vi "ReadParamBinFileFromControlProgram.vi"(0 "Array of Params (in format of control software parmas Typedef) in":T6[](array[typedef]) {"Instrument Calibr"."Psi" format="%#_2f"; "Manual Control"."Y peizo\n [nm]" scale=0.0..30000.0; "Manual Control"."AOM0 \nPower" scale=0.0..1.0; "Manual Control"."X piezo\n [nm]" scale=0.0..30000.0; "Manual Control"."Rotation Control"."freq difference [Hz]" step=0.5; "Manual Control"."Rotation Control"."mean freq  [MHz]\ndefault 39.99" min=0.0 step=0.01; "Manual Control"."Rotation Control"."B amp (0-120)" min=0.0 max=120.0 step=0.1; "Manual Control"."Rotation Control"."A amp (0-120)" min=0.0 max=120.0 step=0.1; "Manual Control"."Rotation Control"."Phase" scale=0.0..360.0; "Manual Control"."trap height\n [nm]" scale=1000.0..7500.0; "TaskIDs"."DAQ tasks"."Px taskID" format="%x"; "TaskIDs"."DAQ tasks"."Py taskID" format="%x"; "TaskIDs"."DAQ tasks"."Pz taskID" format="%x"; "TaskIDs"."DAQ tasks"."AOM taskID" format="%x"; "TaskIDs"."DAQ tasks"."Clock taskID" format="%x"; "TaskIDs"."DAQ tasks"."AI taskID" format="%x"}, 1 "file path in":path, 2 "Ignore HF and XYFTC calibration":bool, 3 "error in":errorcluster) -> (7 "Params out":T1={"Manual Control"={"Rotation Control"={"Phase"=0.0, "A amp (0-120)"=75.0, "B amp (0-120)"=53.3, "mean freq  [MHz]\ndefault 39.99"=40.0, "freq difference [Hz]"=2.0, "Enable A"=TRUE, "Enable B"=TRUE}, "X piezo\n [nm]"=0.0, "Y peizo\n [nm]"=0.0, "-Z piezo\n [nm]"=5.012658227848101, "AOM0 \nPower"=0.2}, "Piezo Calibr"={"Px2Vx(AO)"=nan, "Py2Vy(AO)"=nan, "Pz2Vz(AO)"=nan, "Min Px"=nan, "Min Py"=nan, "Min Pz"=nan, "Max Px"=nan, "Max Py"=nan, "Max Pz"=nan, "Vx0 (V)"=nan, "Vy0 (V)"=nan, "Vz0 (V)"=nan}, "Instrument Calibr"={"Angular compensation coeffs"=[], "TetherCenter"={"TrapX_AO 0 [nm]"=nan, "TrapY_AO 0 [nm]"=nan, "TrapZ_AO 0 [nm]"=nan}, "XYZsignal baseline"={"Xsignal0"=nan, "Ysignal0"=nan, "Zsignal0"=nan, "Zsig slope"=nan, "Z bead0"=nan}, "S and P to Vs0"={"Vs0/P"=1.0, "Vs0/S"=1.0}, "Psi"=0.0, "ePS:eRL drift correlation"={"Interc P"=nan, "Slope P"=nan, "Interc S"=nan, "Slope S"=nan}, "Current piezo volt AO"={"Vpx_AO [V]"=nan, "Vpy_AO [V]"=nan, "Vpz_AO [V]"=nan}}, "Cylinder Calibr"={"ZStiff"=nan, "Zsens"=nan, "AngStiff"=nan, "XStiff"=nan, "Xsens"=nan, "MaxEllip"=nan, "YStiff"=nan, "Ysens"=nan, "FocalShift"=nan, "Sfz"=nan, "1/Sz"=nan, "Stau"=nan, "Sfx"=nan, "1/Sx"=nan, "1/Sang"=nan, "Sfy"=nan, "1/Sy"=nan, "1/focal"=nan}, "DAQParams"={"Buffer size"=nan, "Scanning rate"=nan, "Average"=nan, "Sampling rate"=nan, "set dt"=nan}, "DAQ channel offsets"={"A0 [V]"=0.0, "D0 [V]"=0.0, "P0  [V]"=0.0, "S0 [V]"=0.0, "L0 [V]"=0.0, "R0 [V]"=0.0, "Vpx0 [V]"=0.0, "Vpy0 [V]"=0.0, "Vpz0 [V]"=0.0, "Vsum0 [V]"=0.0, "Vpx_AO0 [V]"=0.0, "Vpy_AO0 [V]"=0.0, "Vpz_AO0 [V]"=0.0}, "Z bead polynomial coeffs"=[nan, nan, nan, nan], "Skip button ref"=refnum, "z bead lookup table"={"z signal"=[], "z bead"=[]}, "SP->power Matrix"=[], "Ms2p"=[], "Mp2s"=[], "Polynomial coeff V_px,y,z 2 position (nm)"=[], "task in"=""} {"Instrument Calibr"."Psi" format="%#_2f"; "Manual Control"."Y peizo\n [nm]" scale=0.0..7000.0; "Manual Control"."AOM0 \nPower" scale=0.0..1.0; "Manual Control"."X piezo\n [nm]" scale=0.0..7000.0; "Manual Control"."Rotation Control"."freq difference [Hz]" step=0.5; "Manual Control"."Rotation Control"."mean freq  [MHz]\ndefault 39.99" min=0.0 step=0.01; "Manual Control"."Rotation Control"."B amp (0-120)" min=0.0 max=120.0 step=0.1; "Manual Control"."Rotation Control"."A amp (0-120)" min=0.0 max=120.0 step=0.1; "Manual Control"."Rotation Control"."Phase" scale=0.0..360.0; "Manual Control"."-Z piezo\n [nm]" scale=1000.0..7000.0}, 8 "file path out":path, 9 "Good?":bool, 10 "error out":errorcluster)   [LabVIEW 2017, in "Initialization.lvlib" / "FileManagement.lvlib"]
uses:
  FileManagement.lvlib
  Param_control program_170907.ctl
  <vilib>/Analysis/Matrix/Datatypes/RealMatrix.ctl
  New Param_170907.ctl
  ManualCtrl.ctl
  CylinderCalibrNew.ctl
  SignalConversion/DAQChannelOffsets.ctl
  <vilib>/Analysis/Matrix/NI_Matrix.lvlib
  Initialization.lvlib
  SignalConversion/SignalConverson.lvlib
panel:
  in  "Control software params as\nData type const":T6={"TaskIDs"={"DAQ tasks"={"Px taskID"=0, "Py taskID"=75, "Pz taskID"=53, "AOM taskID"=40, "Clock taskID"=2, "AI taskID"=0}, "DVEHandle"=refnum}, "Manual Control"={"Rotation Control"={"Phase"=0.0, "A amp (0-120)"=75.0, "B amp (0-120)"=53.3, "mean freq  [MHz]\ndefault 39.99"=40.0, "freq difference [Hz]"=2.0, "Enable A"=TRUE, "Enable B"=TRUE}, "X piezo\n [nm]"=nan, "Y peizo\n [nm]"=nan, "trap height\n [nm]"=nan, "AOM0 \nPower"=nan}, "Piezo Calibr"={"Px2Vx(AO)"=nan, "Py2Vy(AO)"=nan, "Pz2Vz(AO)"=nan, "Min Px"=nan, "Min Py"=0.0, "Min Pz"=nan, "Max Px"=nan, "Max Py"=nan, "Max Pz"=nan, "Vx0 (V)"=nan, "Vy0 (V)"=nan, "Vz0 (V)"=nan}, "Instrument Calibr"={"Angular compensation coeffs"=[], "TetherCenter"={"TrapX_AO 0 [nm]"=nan, "TrapY_AO 0 [nm]"=nan, "TrapZ_AO 0 [nm]"=nan}, "XYZsignal baseline"={"Xsignal0"=nan, "Ysignal0"=nan, "Zsignal0"=nan, "Zsig slope"=nan, "Z bead0"=nan}, "S and P to Vs0"={"Vs0/P"=1.0, "Vs0/S"=1.0}, "Psi"=nan, "ePS:eRL drift correlation"={"Interc P"=nan, "Slope P"=nan, "Interc S"=nan, "Slope S"=nan}, "Current piezo volt AO"={"Vpx_AO [V]"=nan, "Vpy_AO [V]"=nan, "Vpz_AO [V]"=nan}}, "Cylinder Calibr"={"ZStiff"=nan, "Zsens"=nan, "AngStiff"=nan, "XStiff"=nan, "Xsens"=nan, "MaxEllip"=nan, "YStiff"=nan, "Ysens"=nan, "FocalShift"=nan, "Sfz"=nan, "1/Sz"=nan, "Stau"=nan, "Sfx"=nan, "1/Sx"=nan, "1/Sang"=nan, "Sfy"=nan, "1/Sy"=nan, "1/focal"=nan}, "DAQParams"={"Buffer size"=0.0, "Scanning rate"=0.0, "Average"=0.0, "Sampling rate"=0.0, "set dt"=0.0}, "DAQ channel offsets"={"A0 [V]"=0.0, "D0 [V]"=0.0, "P0  [V]"=0.0, "S0 [V]"=0.0, "L0 [V]"=0.0, "R0 [V]"=0.0, "Vpx0 [V]"=0.0, "Vpy0 [V]"=0.0, "Vpz0 [V]"=0.0, "Vsum0 [V]"=0.0, "Vpx_AO0 [V]"=0.0, "Vpy_AO0 [V]"=0.0, "Vpz_AO0 [V]"=0.0}, "Z bead polynomial coeffs"=[nan, nan, nan, nan], "Skip button ref"=refnum, "z bead lookup table"={"z signal"=[], "z bead"=[]}, "SP->power Matrix"=[], "Ms2p"=[], "Mp2s"=[], "Polynomial coeff V_px,y,z 2 position (nm)"=[]} {"Instrument Calibr"."Psi" format="%#_2f"; "Manual Control"."Y peizo\n [nm]" scale=0.0..30000.0; "Manual Control"."AOM0 \nPower" scale=0.0..1.0; "Manual Control"."X piezo\n [nm]" scale=0.0..30000.0; "Manual Control"."Rotation Control"."freq difference [Hz]" step=0.5; "Manual Control"."Rotation Control"."mean freq  [MHz]\ndefault 39.99" min=0.0 step=0.01; "Manual Control"."Rotation Control"."B amp (0-120)" min=0.0 max=120.0 step=0.1; "Manual Control"."Rotation Control"."A amp (0-120)" min=0.0 max=120.0 step=0.1; "Manual Control"."Rotation Control"."Phase" scale=0.0..360.0; "Manual Control"."trap height\n [nm]" scale=1000.0..7500.0; "TaskIDs"."DAQ tasks"."Px taskID" format="%x"; "TaskIDs"."DAQ tasks"."Py taskID" format="%x"; "TaskIDs"."DAQ tasks"."Pz taskID" format="%x"; "TaskIDs"."DAQ tasks"."AOM taskID" format="%x"; "TaskIDs"."DAQ tasks"."Clock taskID" format="%x"; "TaskIDs"."DAQ tasks"."AI taskID" format="%x"}
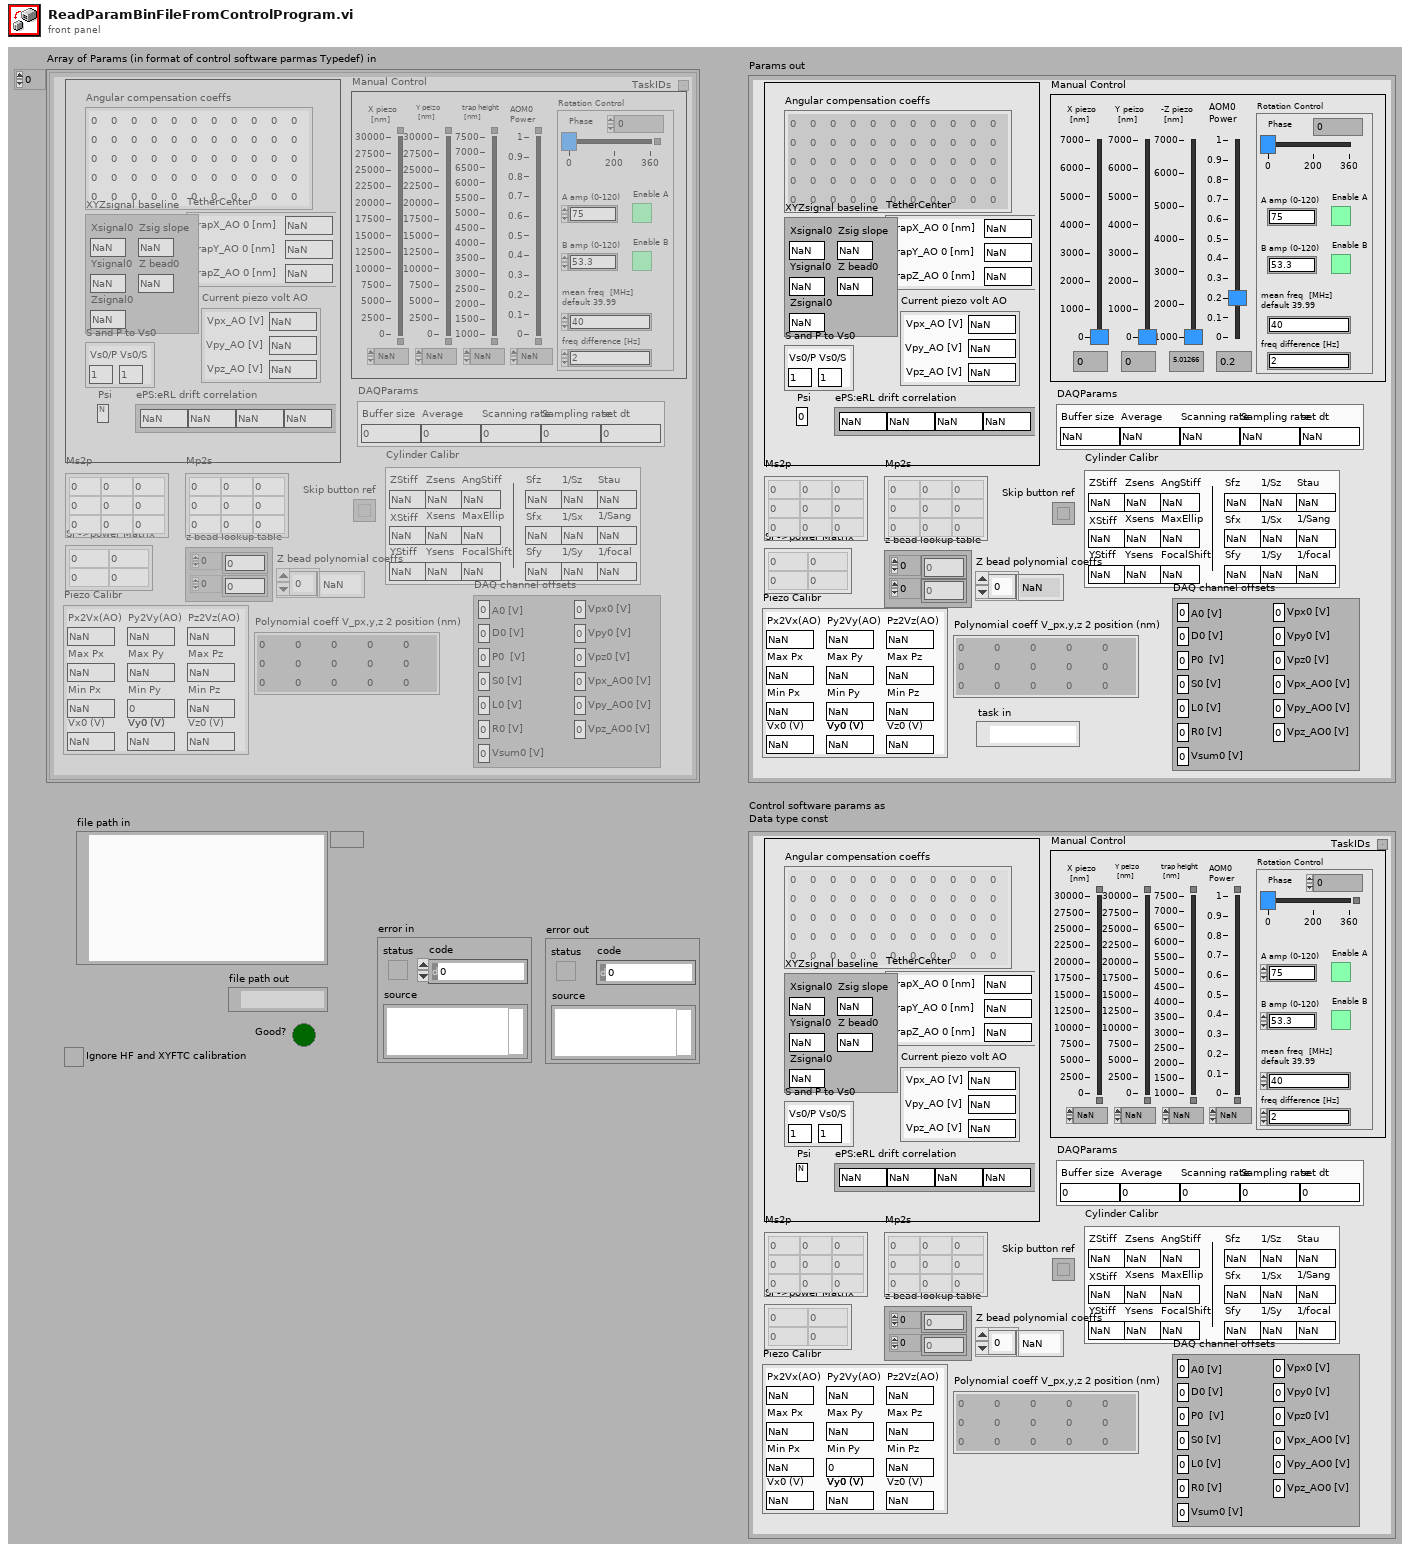
[diagram p1: front panel]
types:
  T1 = typedef "Initialization.lvlib/New Param_170907.ctl" = cluster{"Manual Control":T2, "Piezo Calibr":cluster{"Px2Vx(AO)":dbl, "Py2Vy(AO)":dbl, "Pz2Vz(AO)":dbl, "Min Px":dbl, "Min Py":dbl, "Min Pz":dbl, "Max Px":dbl, "Max Py":dbl, "Max Pz":dbl, "Vx0 (V)":dbl, "Vy0 (V)":dbl, "Vz0 (V)":dbl}, "Instrument Calibr":cluster{"Angular compensation coeffs":dbl[][], "TetherCenter":cluster{"TrapX_AO 0 [nm]":dbl, "TrapY_AO 0 [nm]":dbl, "TrapZ_AO 0 [nm]":dbl}, "XYZsignal baseline":cluster{"Xsignal0":dbl, "Ysignal0":dbl, "Zsignal0":dbl, "Zsig slope":dbl, "Z bead0":dbl}, "S and P to Vs0":cluster{"Vs0/P":dbl, "Vs0/S":dbl}, "Psi":dbl, "ePS:eRL drift correlation":cluster{"Interc P":dbl, "Slope P":dbl, "Interc S":dbl, "Slope S":dbl}, "Current piezo volt AO":cluster{"Vpx_AO [V]":dbl, "Vpy_AO [V]":dbl, "Vpz_AO [V]":dbl}}, "Cylinder Calibr":T3, "DAQParams":cluster{"Buffer size":dbl, "Scanning rate":dbl, "Average":dbl, "Sampling rate":dbl, "set dt":dbl}, "DAQ channel offsets":T4, "Z bead polynomial coeffs":dbl[], "Skip button ref":refnum<vi>, "z bead lookup table":cluster{"z signal":dbl[], "z bead":dbl[]}, "SP->power Matrix":T5, "Ms2p":T5, "Mp2s":T5, "Polynomial coeff V_px,y,z 2 position (nm)":dbl[][], "task in":refnum<k21>}
  T2 = typedef "Initialization.lvlib/ManualCtrl.ctl" = cluster{"Rotation Control":cluster{"Phase":dbl, "A amp (0-120)":dbl, "B amp (0-120)":dbl, "mean freq  [MHz]\ndefault 39.99":dbl, "freq difference [Hz]":dbl, "Enable A":bool, "Enable B":bool}, "X piezo\n [nm]":dbl, "Y peizo\n [nm]":dbl, "-Z piezo\n [nm]":dbl, "AOM0 \nPower":dbl}
  T3 = typedef "Initialization.lvlib/CylinderCalibrNew.ctl" = cluster{"ZStiff":dbl, "Zsens":dbl, "AngStiff":dbl, "XStiff":dbl, "Xsens":dbl, "MaxEllip":dbl, "YStiff":dbl, "Ysens":dbl, "FocalShift":dbl, "Sfz":dbl, "1/Sz":dbl, "Stau":dbl, "Sfx":dbl, "1/Sx":dbl, "1/Sang":dbl, "Sfy":dbl, "1/Sy":dbl, "1/focal":dbl}
  T4 = typedef "SignalConverson.lvlib/DAQChannelOffsets.ctl" = cluster{"A0 [V]":dbl, "D0 [V]":dbl, "P0  [V]":dbl, "S0 [V]":dbl, "L0 [V]":dbl, "R0 [V]":dbl, "Vpx0 [V]":dbl, "Vpy0 [V]":dbl, "Vpz0 [V]":dbl, "Vsum0 [V]":dbl, "Vpx_AO0 [V]":dbl, "Vpy_AO0 [V]":dbl, "Vpz_AO0 [V]":dbl}
  T5 = typedef "NI_Matrix.lvlib/RealMatrix.ctl" = dbl[][]
  T6 = typedef "Initialization.lvlib/Param_control program_170907.ctl" = cluster{"TaskIDs":cluster{"DAQ tasks":cluster{"Px taskID":u32, "Py taskID":u32, "Pz taskID":u32, "AOM taskID":u32, "Clock taskID":u32, "AI taskID":u32}, "DVEHandle":refnum<file>}, "Manual Control":cluster{"Rotation Control":cluster{"Phase":dbl, "A amp (0-120)":dbl, "B amp (0-120)":dbl, "mean freq  [MHz]\ndefault 39.99":dbl, "freq difference [Hz]":dbl, "Enable A":bool, "Enable B":bool}, "X piezo\n [nm]":dbl, "Y peizo\n [nm]":dbl, "trap height\n [nm]":dbl, "AOM0 \nPower":dbl}, "Piezo Calibr":cluster{"Px2Vx(AO)":dbl, "Py2Vy(AO)":dbl, "Pz2Vz(AO)":dbl, "Min Px":dbl, "Min Py":dbl, "Min Pz":dbl, "Max Px":dbl, "Max Py":dbl, "Max Pz":dbl, "Vx0 (V)":dbl, "Vy0 (V)":dbl, "Vz0 (V)":dbl}, "Instrument Calibr":cluster{"Angular compensation coeffs":dbl[][], "TetherCenter":cluster{"TrapX_AO 0 [nm]":dbl, "TrapY_AO 0 [nm]":dbl, "TrapZ_AO 0 [nm]":dbl}, "XYZsignal baseline":cluster{"Xsignal0":dbl, "Ysignal0":dbl, "Zsignal0":dbl, "Zsig slope":dbl, "Z bead0":dbl}, "S and P to Vs0":cluster{"Vs0/P":dbl, "Vs0/S":dbl}, "Psi":dbl, "ePS:eRL drift correlation":cluster{"Interc P":dbl, "Slope P":dbl, "Interc S":dbl, "Slope S":dbl}, "Current piezo volt AO":cluster{"Vpx_AO [V]":dbl, "Vpy_AO [V]":dbl, "Vpz_AO [V]":dbl}}, "Cylinder Calibr":cluster{"ZStiff":dbl, "Zsens":dbl, "AngStiff":dbl, "XStiff":dbl, "Xsens":dbl, "MaxEllip":dbl, "YStiff":dbl, "Ysens":dbl, "FocalShift":dbl, "Sfz":dbl, "1/Sz":dbl, "Stau":dbl, "Sfx":dbl, "1/Sx":dbl, "1/Sang":dbl, "Sfy":dbl, "1/Sy":dbl, "1/focal":dbl}, "DAQParams":cluster{"Buffer size":dbl, "Scanning rate":dbl, "Average":dbl, "Sampling rate":dbl, "set dt":dbl}, "DAQ channel offsets":cluster{"A0 [V]":dbl, "D0 [V]":dbl, "P0  [V]":dbl, "S0 [V]":dbl, "L0 [V]":dbl, "R0 [V]":dbl, "Vpx0 [V]":dbl, "Vpy0 [V]":dbl, "Vpz0 [V]":dbl, "Vsum0 [V]":dbl, "Vpx_AO0 [V]":dbl, "Vpy_AO0 [V]":dbl, "Vpz_AO0 [V]":dbl}, "Z bead polynomial coeffs":dbl[], "Skip button ref":refnum<vi>, "z bead lookup table":cluster{"z signal":dbl[], "z bead":dbl[]}, "SP->power Matrix":T5, "Ms2p":T5, "Mp2s":T5, "Polynomial coeff V_px,y,z 2 position (nm)":dbl[][]}
  T7 = enum16{"open", "replace", "create", "open or create", "replace or create", "replace or create with confirmation"}
  T8 = cluster{"Rotation Control":cluster{"Phase":dbl, "A amp (0-120)":dbl, "B amp (0-120)":dbl, "mean freq  [MHz]\ndefault 39.99":dbl, "freq difference [Hz]":dbl, "Enable A":bool, "Enable B":bool}, "X piezo\n [nm]":dbl, "Y peizo\n [nm]":dbl, "trap height\n [nm]":dbl, "AOM0 \nPower":dbl}
  T9 = cluster{"Px2Vx(AO)":dbl, "Py2Vy(AO)":dbl, "Pz2Vz(AO)":dbl, "Min Px":dbl, "Min Py":dbl, "Min Pz":dbl, "Max Px":dbl, "Max Py":dbl, "Max Pz":dbl, "Vx0 (V)":dbl, "Vy0 (V)":dbl, "Vz0 (V)":dbl}
  T10 = cluster{"Angular compensation coeffs":dbl[][], "TetherCenter":cluster{"TrapX_AO 0 [nm]":dbl, "TrapY_AO 0 [nm]":dbl, "TrapZ_AO 0 [nm]":dbl}, "XYZsignal baseline":cluster{"Xsignal0":dbl, "Ysignal0":dbl, "Zsignal0":dbl, "Zsig slope":dbl, "Z bead0":dbl}, "S and P to Vs0":cluster{"Vs0/P":dbl, "Vs0/S":dbl}, "Psi":dbl, "ePS:eRL drift correlation":cluster{"Interc P":dbl, "Slope P":dbl, "Interc S":dbl, "Slope S":dbl}, "Current piezo volt AO":cluster{"Vpx_AO [V]":dbl, "Vpy_AO [V]":dbl, "Vpz_AO [V]":dbl}}
  T11 = cluster{"ZStiff":dbl, "Zsens":dbl, "AngStiff":dbl, "XStiff":dbl, "Xsens":dbl, "MaxEllip":dbl, "YStiff":dbl, "Ysens":dbl, "FocalShift":dbl, "Sfz":dbl, "1/Sz":dbl, "Stau":dbl, "Sfx":dbl, "1/Sx":dbl, "1/Sang":dbl, "Sfy":dbl, "1/Sy":dbl, "1/focal":dbl}
  T12 = cluster{"Buffer size":dbl, "Scanning rate":dbl, "Average":dbl, "Sampling rate":dbl, "set dt":dbl}
  T13 = cluster{"A0 [V]":dbl, "D0 [V]":dbl, "P0  [V]":dbl, "S0 [V]":dbl, "L0 [V]":dbl, "R0 [V]":dbl, "Vpx0 [V]":dbl, "Vpy0 [V]":dbl, "Vpz0 [V]":dbl, "Vsum0 [V]":dbl, "Vpx_AO0 [V]":dbl, "Vpy_AO0 [V]":dbl, "Vpz_AO0 [V]":dbl}
  T14 = cluster{"TrapX_AO 0 [nm]":dbl, "TrapY_AO 0 [nm]":dbl, "TrapZ_AO 0 [nm]":dbl}
  T15 = cluster{"Xsignal0":dbl, "Ysignal0":dbl, "Zsignal0":dbl, "Zsig slope":dbl, "Z bead0":dbl}
  T16 = cluster{"Interc P":dbl, "Slope P":dbl, "Interc S":dbl, "Slope S":dbl}
  T17 = cluster{"Vpx_AO [V]":dbl, "Vpy_AO [V]":dbl, "Vpz_AO [V]":dbl}
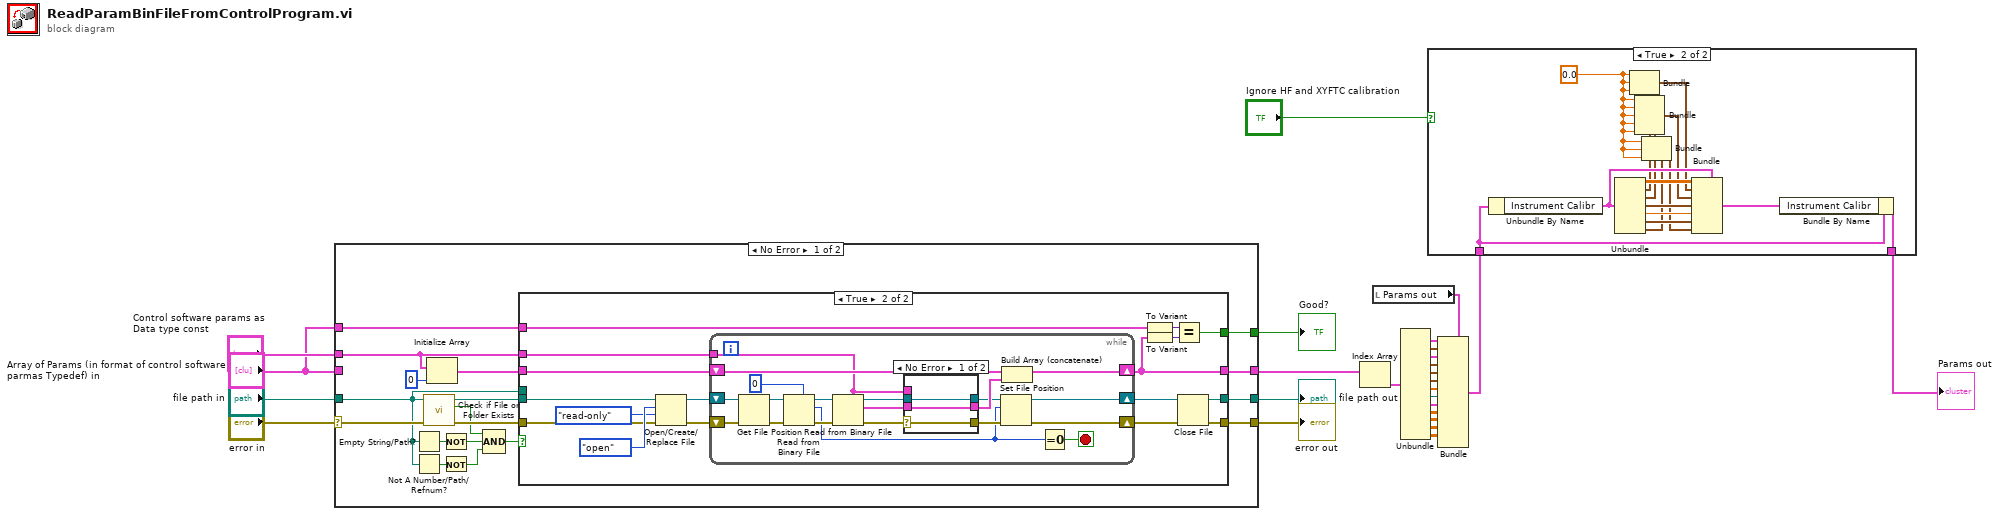
[diagram p0: block diagram]
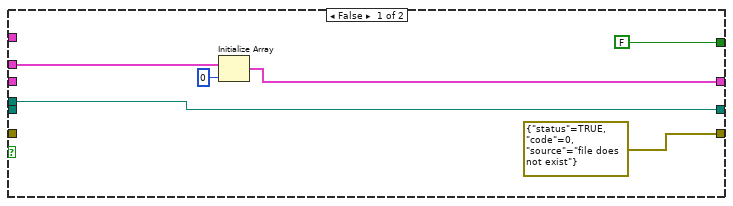
[diagram p3: hidden frame]
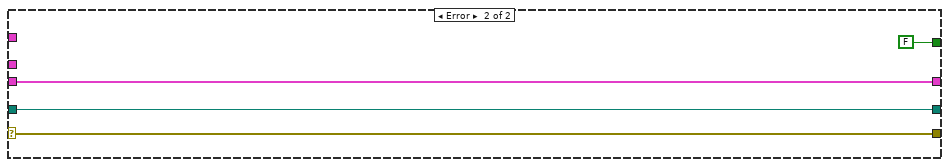
[diagram p5: hidden frame]
diagram:
  n1 = case shown="No Error" "error in" {
    selector: "error in" -> [w38 w96]
    tunnel: "file path in" -> [w31 w95]
    tunnel: "Array of Params (in format of control software parmas Typedef) in" -> [_ w94]
    tunnel: [w44 w96] -> w26
    tunnel: [w43 w95] -> w25
    tunnel: [w42 w94] -> w19
    tunnel: "Control software params as\nData type const" -> [w41 _]
    tunnel: "Array of Params (in format of control software parmas Typedef) in" -> [w40 _]
    tunnel: [w39 FALSE] -> w23
    frame No Error {
      n2 = Empty String/Path?(string/path=w31) -> (empty?=w33:bool)
      n3 = Not A Number/Path/Refnum?(number/path/refnum=w31) -> (NaN/Path/Refnum?=w32:bool)
      n4 = call <vilib>:"Check if File or Folder Exists.vi"("error in (no error)"=w38, "path"=w31) -> ("error out"=w34:errorcluster, "file or folder exists?"=w29:bool, "dup path"=w35:path)  [unwired: 7 in]
      n5 = Initialize Array(w41, 0 ("dimension size")) -> (w36:T6[])
      n6 = Not(x=w33) -> (.not. x?=w28:bool)
      n7 = Not(x=w32) -> (.not. x?=w27:bool)
      n8 = Compound Arithmetic op=AND(w29, w28, w27) -> (w30:bool)
      n9 = case shown="True" w30 {
        tunnel: [w48 w63] -> w42
        tunnel: w41 -> [w49 w67]
        tunnel: [w45 w58] -> w43
        tunnel: [errorcluster {"status"=TRUE, "code"=0, "source"="file does not exist"} ("error out") w59] -> w44
        tunnel: w36 -> [_ w66]
        tunnel: w40 -> [_ w62]
        tunnel: [FALSE w61] -> w39
        tunnel: w31 -> [w45 _]
        tunnel: w35 -> [_ w52]
        tunnel: w34 -> [_ w51]
        frame False {
          n10 = Initialize Array(w49, 0 ("dimension size")) -> (w48:T6[])
        }
        frame True {
          n11 = Open/Create/Replace File(file path (use dialog)=w52, error in=w51, operation (0:open)=T7."open", access (0:read/write)=enum16{"read/write", "read-only", "write-only"}."read-only") -> (refnum out=w53:refnum<file>, error out=w54:errorcluster)  [unwired: 2 in, 1 out]
          n12 = while {
            shift-right: [w86] -> w63
            shift-left: w66 -> [w84]
            tunnel: w67 -> [w69]
            shift-right: [w73] -> w57
            shift-left: w53 -> [w78]
            shift-right: [w72] -> w60
            shift-left: w54 -> [w81]
            stop <- w87 stop-if-true
            n13 = Get File Position(4:w81, 7:w78) -> (0:w80:errorcluster, 3:w79:refnum<file>)  [unwired: 1 out]
            n14 = Read from Binary File(5:i64 0, 8:w80, 11:w79) -> (0:w82:errorcluster, 2:w68:i64, 3:w83:refnum<file>)  [unwired: 3 in, 1 out]
            n15 = Read from Binary File(5:w69, 8:w82, 11:w83) -> (0:w76:errorcluster, 2:w75:T6, 3:w77:refnum<file>)  [unwired: 3 in, 1 out]
            n16 = case shown="No Error" w76 {
              selector: w76 -> [w89 _]
              tunnel: w77 -> [w88 w91]
              tunnel: w75 -> [w90 _]
              tunnel: [w90 w92] -> w74
              tunnel: [w89 _] -> w71
              tunnel: [w88 w91] -> w70
              tunnel: w69 -> [_ w92]
              frame No Error {
              }
              frame Error {
              }
            }
            n17 = Set File Position(offset (in bytes) (0)=w68, refnum=w70, error in=w71) -> (refnum out=w73:refnum<file>, error out=w72:errorcluster)  [unwired: 1 in]
            n18 = Build Array (concatenate)(w84, w74) -> (w86:T6[])
            n19 = Equal To 0?(x=w68) -> (x = 0?=w87:bool)
          }
          n20 = To Variant(anything=w62) -> (Variant=w65:variant)
          n21 = To Variant(anything=w63) -> (Variant=w64:variant)
          n22 = Equal?(x=w65, y=w64) -> (x = y?=w61:bool)
          n23 = Close File(refnum=w57, error in=w60) -> (path=w58:path, error out=w59:errorcluster)
        }
      }
    }
    frame Error {
    }
  }
  "error out" <- w26
  "file path out" <- w25
  "Good?" <- w23
  n24 = Index Array(array=w19) -> (element=w18:T6)  [unwired: 1 in]
  n25 = local read "Params out"() -> (w17:T1)
  n26 = Unbundle(w18) -> ("Manual Control"=w4:T8, "Piezo Calibr"=w5:T9, "Instrument Calibr"=w6:T10, "Cylinder Calibr"=w7:T11, "DAQParams"=w8:T12, "DAQ channel offsets"=w9:T13, "Z bead polynomial coeffs"=w10:dbl[], "Skip button ref"=w11:refnum<vi>, "z bead lookup table"=w12:cluster{"z signal":dbl[], "z bead":dbl[]}, "SP->power Matrix"=w13:T5, "Ms2p"=w14:T5, "Mp2s"=w15:T5, "Polynomial coeff V_px,y,z 2 position (nm)"=w16:dbl[][])  [unwired: 1 out]
  n27 = Bundle(cluster=w17, "Manual Control"=w4, "Piezo Calibr"=w5, "Instrument Calibr"=w6, "Cylinder Calibr"=w7, "DAQParams"=w8, "DAQ channel offsets"=w9, "Z bead polynomial coeffs"=w10, "Skip button ref"=w11, "z bead lookup table"=w12, "SP->power Matrix"=w13, "Ms2p"=w14, "Mp2s"=w15, "Polynomial coeff V_px,y,z 2 position (nm)"=w16) -> (w3:T1)  [unwired: 1 in]
  n28 = case shown="True" "Ignore HF and XYFTC calibration" {
    tunnel: w3 -> [w97 w100]
    tunnel: [w97 w99] -> w2
    frame False {
    }
    frame True {
      w101 = 0.0
      n29 = Unbundle By Name(w100) -> ("Instrument Calibr"=w112:T10)
      n30 = Unbundle(w112) -> ("Angular compensation coeffs"=w111:dbl[][], "TetherCenter"=w110:T14, "XYZsignal baseline"=w108:T15, "S and P to Vs0"=w106:cluster{"Vs0/P":dbl, "Vs0/S":dbl}, "Psi"=w105:dbl, "ePS:eRL drift correlation"=w104:T16, "Current piezo volt AO"=w103:T17)
      n31 = Bundle(cluster=w110, "TrapX_AO 0 [nm]"=w101, "TrapY_AO 0 [nm]"=w101, "TrapZ_AO 0 [nm]"=w101) -> (w109:T14)
      n32 = Bundle(cluster=w108, "Xsignal0"=w101, "Ysignal0"=w101, "Zsignal0"=w101, "Zsig slope"=w101, "Z bead0"=w101) -> (w107:T15)
      n33 = Bundle(cluster=w103, "Vpx_AO [V]"=w101, "Vpy_AO [V]"=w101, "Vpz_AO [V]"=w101) -> (w102:T17)
      n34 = Bundle(cluster=w112, "Angular compensation coeffs"=w111, "TetherCenter"=w109, "XYZsignal baseline"=w107, "S and P to Vs0"=w106, "Psi"=w105, "ePS:eRL drift correlation"=w104, "Current piezo volt AO"=w102) -> (w98:T10)
      n35 = Bundle By Name(cluster=w100, "Instrument Calibr"=w98) -> (w99:T1)
    }
  }
  "Params out" <- w2
